vi "Read Listbox Header (UTF-8 String).vi"(8 "error in":errorcluster, 11 "Control Ref":refnum<vi>) -> (0 "error out":errorcluster, 2 "Value":refnum<class "UTF-8 String.lvclass">)   [LabVIEW 2020, in "G-Unicode.lvlib"]
doc: "Read unicode text from a control or text element of a control. If the control text is not unicode, it will be converted to unicode."
uses:
  G-Unicode.lvlib
  Types/UTF-8 String/UTF-8 String.lvclass
  Types/UTF-8 String/UTF-8 String.lvclass/UTF-8 String.ctl
  bfba3187-b22e-4285-8cc2-1816a803f974.vi
  Types/UTF-8 String/New UTF-8 String.vi
  Unicode/Encode String.vi
  Private/Conversion/Text to UTF-8.vi
  Private/Conversion/Polymorphic VIs/Text to UTF-8 (LabVIEW String).vi
  Private/Conversion/Encoded UTF-8 String to Encoded UTF-16LE String.vi
  Unicode/SubVIs/UTF-16 Byte Swap.vi
  Private/Conversion/UTF-8 to Text.vi
  Private/Conversion/Polymorphic VIs/UTF-8 to Text (LabVIEW String).vi
  Private/Conversion/Encoded UTF-16LE String to Encoded UTF-8 String.vi
  Unicode/Prepend BOM.vi
  Unicode/SubVIs/Byte Order Marks.vi
  Unicode/Detect BOM.vi
  Unicode/Detect String Encoding.vi
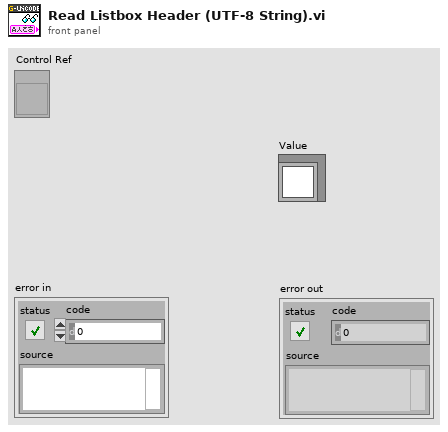
[diagram p1: front panel]
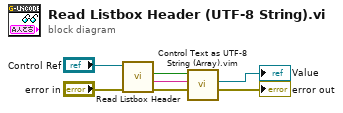
[diagram p0: block diagram]
diagram:
  n1 = call "Read Listbox Header.vi"("error in"="error in", "Listbox Ref in"="Control Ref") -> ("error out"=w3:errorcluster, "Value"=w5:string, "Interpret As Unicode"=w6:bool)  [unwired: 6 in, 1 out]
  n2 = call "Control Text as UTF-8 String (Array).vim"("Interpret As Unicode"=w6, "error in"=w3, "Control Text"=w5) -> ("error out"=→"error out":errorcluster, "UTF-8 String"=→"Value":refnum<class "UTF-8 String.lvclass">)  [unwired: 7 in]
